vi "Configure.vi"(8 "error in (no error)":errorcluster, 11 "Trace in":refnum<class "Trace.lvclass">) -> (0 "error out":errorcluster, 2 "cancelled?":bool, 3 "Trace out":refnum<class "Trace.lvclass">)   [LabVIEW 2012, in "Trace.lvclass"]
doc: "The configure method configures the details for the RabbitMQ connection, the observers and the mapping script.\n\nIn the derived class, make a call to the parent for setting these parameters."
uses:
  Trace.lvclass
  <vilib>/Distrio/Murmex/Murmex/Murmex.lvclass
panel:
  # "RabbitMQ parameters"
  # "Window position"
  # "Sends a setting or configuration value to an observer, e.g. observer.parameter=settingsname;"
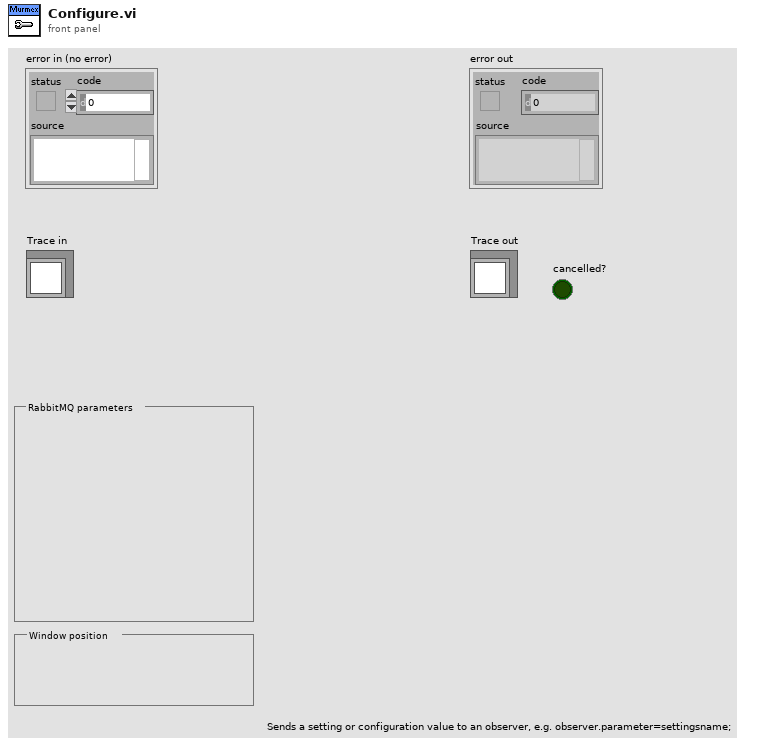
[diagram p1: front panel]
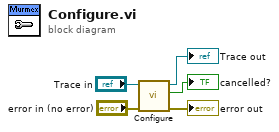
[diagram p0: block diagram]
diagram:
  n1 = call-parent "Configure.vi"("error in (no error)"="error in (no error)", "Murmex in"="Trace in") -> ("error out"=→"error out":errorcluster, "cancelled?"=→"cancelled?":bool, "Murmex out"=→"Trace out":refnum<class "Trace.lvclass">)  [unwired: 7 in]
